vi "SeCrTs-AO_Write.vi"(7 "Data FIFO Ref":T1, 8 "error in (no error)":errorcluster, 10 "AO_Task":refnum<k21>) -> (0 "error out":errorcluster, 2 "task out":refnum<k21>)   [LabVIEW 2022 SP3]
uses:
  RT Controls/SeCrTs-Data FIFO.ctl
  <vilib>/Platform/TimedLoop/XDataNode/timing_clust.ctl
  <vilib>/Platform/TimedLoop/XDataNode/nitl_modes.ctl
  <vilib>/Platform/TimedLoop/XDataNode/wakeup.ctl
  <vilib>/DAQmx/write.llb/DAQmx Write (Analog DBL 1Chan 1Samp).vi
  <vilib>/DAQmx/miscellaneous.llb/DAQmx Fill In Error Info.vi
  <vilib>/platform/TimedLoop/XDataNode/XDataNode.xnode
  <vilib>/Platform/TimedLoop/XDataNode/XDNodeRunTimeDep.lvlib
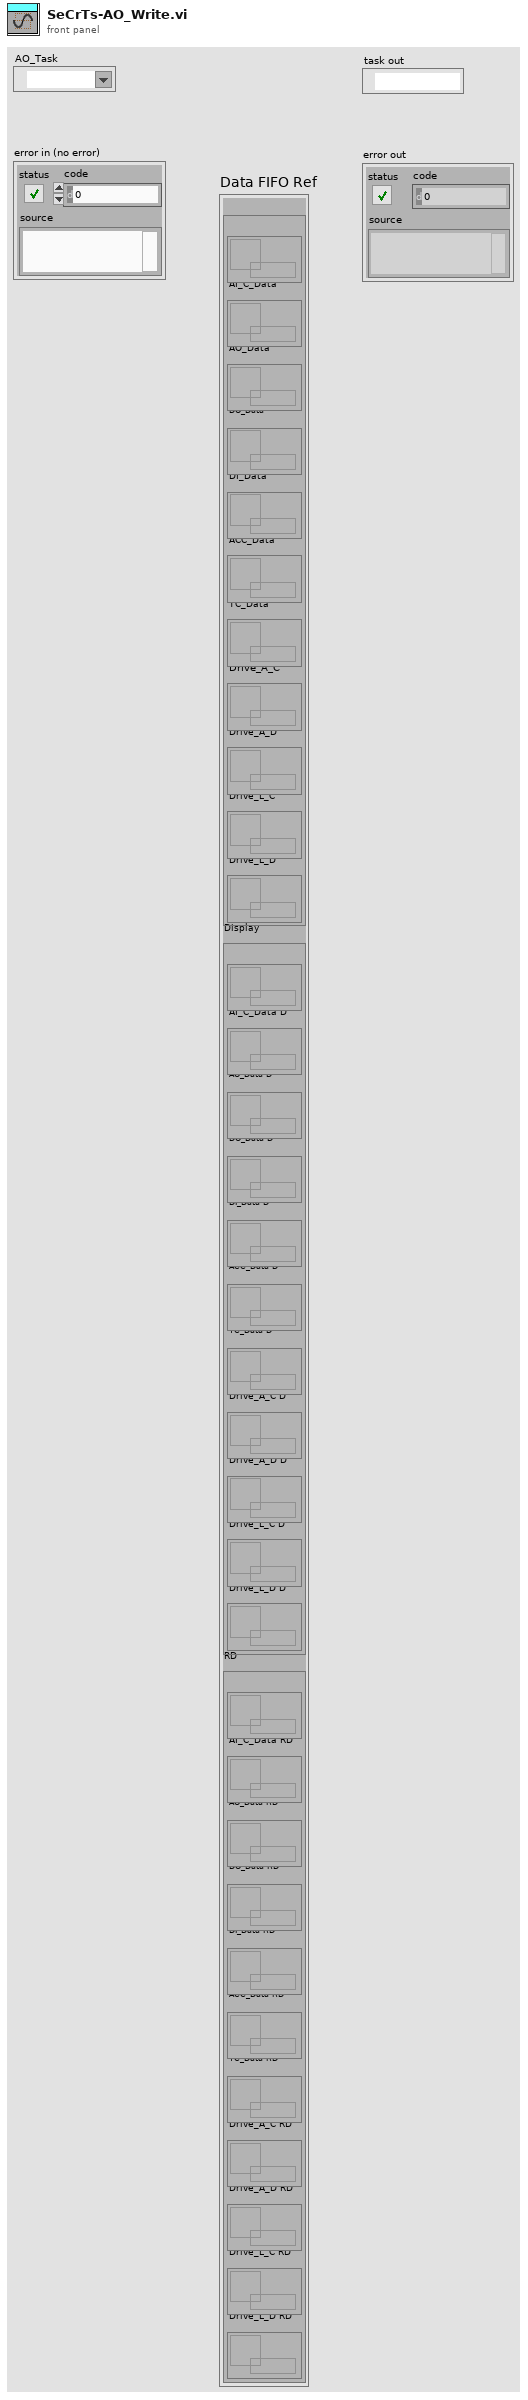
[diagram p1: front panel]
types:
  T1 = typedef "SeCrTs-Data FIFO.ctl" = cluster{"Control":cluster{"AI_V_Data":refnum<queue>, "AI_C_Data":refnum<queue>, "AO_Data":refnum<queue>, "DO_Data":refnum<queue>, "DI_Data":refnum<queue>, "ACC_Data":refnum<queue>, "TC_Data":refnum<queue>, "Drive_A_C":refnum<queue>, "Drive_A_D":refnum<queue>, "Drive_L_C":refnum<queue>, "Drive_L_D":refnum<queue>}, "Display":cluster{"AI_V_Data D":refnum<queue>, "AI_C_Data D":refnum<queue>, "AO_Data D":refnum<queue>, "DO_Data D":refnum<queue>, "DI_Data D":refnum<queue>, "ACC_Data D":refnum<queue>, "TC_Data D":refnum<queue>, "Drive_A_C D":refnum<queue>, "Drive_A_D D":refnum<queue>, "Drive_L_C D":refnum<queue>, "Drive_L_D D":refnum<queue>}, "RD":cluster{"AI_V_Data RD":refnum<queue>, "AI_C_Data RD":refnum<queue>, "AO_Data RD":refnum<queue>, "DO_Data RD":refnum<queue>, "DI_Data RD":refnum<queue>, "ACC_Data RD":refnum<queue>, "TC_Data RD":refnum<queue>, "Drive_A_C RD":refnum<queue>, "Drive_A_D RD":refnum<queue>, "Drive_L_C RD":refnum<queue>, "Drive_L_D RD":refnum<queue>}}
  T2 = typedef "XDNodeRunTimeDep.lvlib/timing_clust.ctl" = cluster{"Expected End [f-1]":u64, "Actual End [f-1]":u64, "Finished Late? [f-1]":bool, "Expected End [i-1]":u64, "Actual End [i-1]":u64, "Finished Late? [i-1]":bool, "Expected Start [i]":u64, "Actual Start [i]":u64, "Expected Start [f]":u64, "Actual Start [f]":u64, "Source Name":string, "Structure Name":string, "Period":i64, "Deadline":i64, "Offset":i64, "Start":i64, "Priority":i32, "Timeout":i32, "Mode":T3, "Wakeup Reason":T4, "Error":errorcluster, "Source Type":string, "Secondary Source Type":string, "Global End Time":u64, "Global Start Time":u64, "Frame Duration":u64, "Iteration Duration":u64, "Assigned CPU":i32, "I/O Scan Engine Mode":u32}
  T3 = typedef "XDNodeRunTimeDep.lvlib/nitl_modes.ctl" = enum32{"No Change", "Process missed periods, maintain original phase", "Discard missed periods, maintain original phase", "Process missed periods, ignore original phase", "Discard missed periods, ignore original phase"}
  T4 = typedef "XDNodeRunTimeDep.lvlib/wakeup.ctl" = enum32{"Normal", "Aborted", "Asynchronous wakeup", "Timing source error", "Timed loop error", "Timeout"}
  T5 = enum16{"AI C", "AI V", "AO", "DI", "DO", "TC", "ACC", "DR L", "DR A"}
  T6 = enum16{"Init", "Read 'All'", "Read 'n'", "Read '1'", "Write '1'", "Write 'n'", "Write 'All'"}
  T7 = cluster{"Start DAQ":bool, "Stop DAQ":bool, "RT Stop":bool, "RT Exit":bool, "Start Seq":bool}
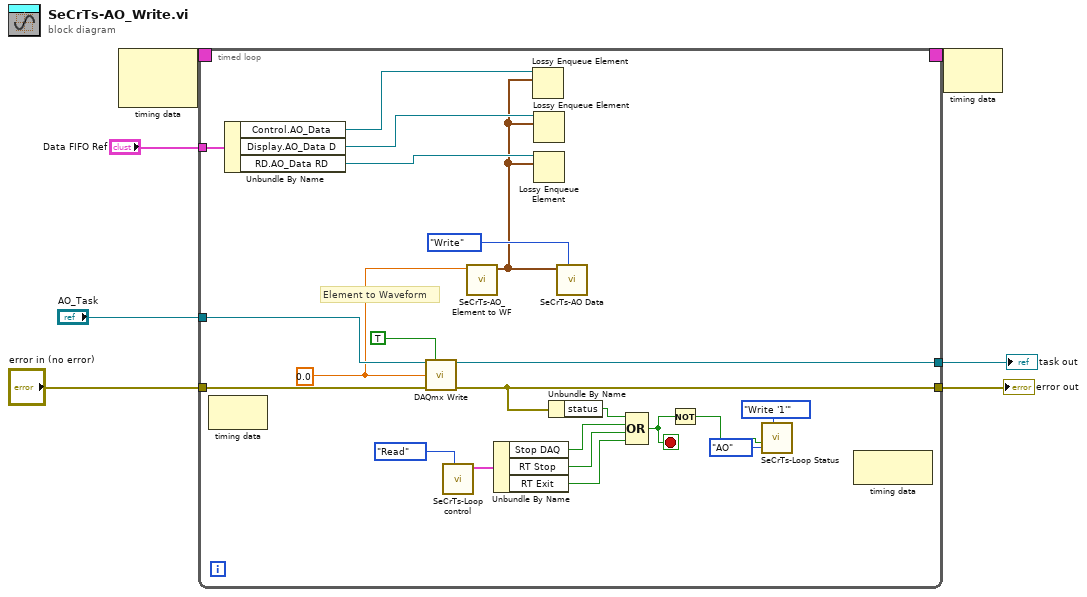
[diagram p0: block diagram]
diagram:
  n1 = node-c288() -> (w7:T2)  [unwired: 2 in]
  n2 = timed-loop {
    tunnel: [w29] -> w2
    tunnel: "AO_Task" -> [w27]
    tunnel: "error in (no error)" -> [w26]
    tunnel: [w23] -> w5
    timing: w7 -> [_]
    timing-out: [_] -> w6
    tunnel: "Data FIFO Ref" -> [w16]
    stop <- w24 stop-if-true
    w11 = 0.0 ("data")
    # "Element to Waveform"
    n3 = node-c288() -> ()  [unwired: 1 in, 1 out]
    n4 = Unbundle By Name(w16) -> ("Control.AO_Data"=w15:refnum<queue>, "Display.AO_Data D"=w14:refnum<queue>, "RD.AO_Data RD"=w13:refnum<queue>)
    n5 = call-poly <vilib>:"DAQmx Write.vi"("task/channels in"=w27, "auto start"=TRUE, "data"=w11, "error in"=w26) -> ("task out"=w23:refnum<k21>, "error out"=w29:errorcluster)  [unwired: 9 in, 1 out]
    n6 = call "SeCrTs-Loop control.vi"("Action"=enum16{"Init", "Write", "Read"}."Read") -> ("Loop Control out"=w21:T7)  [unwired: 9 in, 1 out]
    n7 = call "SeCrTs-AO_Element to WF.vi"("AO Array"=w11) -> ("Array"=w12:waveform(dbl)[])  [unwired: 10 in]
    n8 = Unbundle By Name(w21) -> ("Stop DAQ"=w20:bool, "RT Stop"=w19:bool, "RT Exit"=w18:bool)
    n9 = Lossy Enqueue Element(queue=w15, element=w12) -> ()  [unwired: 1 in, 4 out]
    n10 = Lossy Enqueue Element(queue=w14, element=w12) -> ()  [unwired: 1 in, 4 out]
    n11 = Lossy Enqueue Element(queue=w13, element=w12) -> ()  [unwired: 1 in, 4 out]
    n12 = Unbundle By Name(w29) -> ("status"=w25:bool)
    n13 = call "SeCrTs-AO Data.vi"("Enum"=enum16{"Write", "Read"}."Write", "In_DO data"=w12) -> ()  [unwired: 9 in, 1 out]
    n14 = Compound Arithmetic op=OR(w25, w20, w19, w18) -> (w24:bool)
    n15 = Not(x=w24) -> (.not. x?=w8:bool)
    n16 = call "SeCrTs-Loop Status.vi"("Option"=T6."Write '1'", "Status"=w8, "Loop"=T5."AO") -> ()  [unwired: 6 in, 3 out]
    n17 = node-c288() -> ()  [unwired: 1 in, 1 out]
  }
  "task out" <- w5
  "error out" <- w2
  n18 = node-c288(w6) -> ()  [unwired: 1 out]
